vi "save.vi"(5 "Control Camera Properties 3":T2={"Packet Size"=1500, "Pixel Format"=17825797, "Gain in dB"=1.0, "Exposure Time in µs"=1500, "Stream Bytes per Second"=50000017} caption="Control Camera Properties" {"Stream Bytes per Second" min=1000000 max=124000000 step=100000 format="%.1p"; "Exposure Time in µs" min=21 max=153391689 format="%#.0f"; "Gain in dB" min=0.0 max=26.0 format="%#_2g"; "Pixel Format" items=["Mono 12 Packed"=17563654, "Mono 12"=17825797]}, 7 "Camera":T1, 8 "Path":path=path "C:/Users/loa/Documents/imaging-spectrometer/imaging-spectrometer/sub_vis/test", 9 "Complete File Name In":string, 10 "Array":u16[][](array[numeric]), 11 "reference":refnum<vi>) -> (0 "saving error out":errorcluster, 1 "Path out":path)   [LabVIEW 2014]
uses:
  type definitions/control camera properties.ctl
  <vilib>/Utility/file.llb/Write To Spreadsheet File (I64).vi
panel:
  # "Bytes"
  # "Trigger"
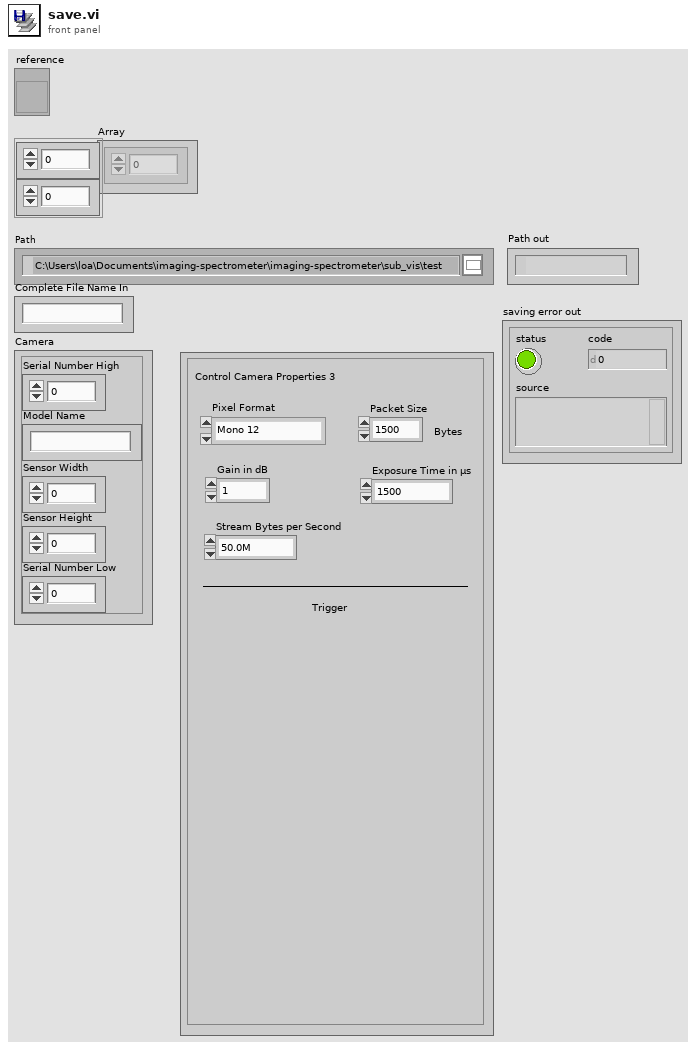
[diagram p1: front panel]
types:
  T1 = cluster{"Serial Number High":u32, "Model Name":string, "Sensor Width":u32, "Sensor Height":u32, "Serial Number Low":u32}
  T2 = typedef "control camera properties.ctl" = cluster{"Packet Size":u32, "Pixel Format":u32, "Gain in dB":dbl, "Exposure Time in µs":u32, "Stream Bytes per Second":u32}
  T3 = enum16{"open", "replace", "create", "open or create", "replace or create", "replace or create with confirmation"}
  T4 = typedef "imagedata.ctl" = cluster{"image type":i32, "image depth":i32, "image":u8[], "mask":u8[], "colors":u32[], "Rectangle":cluster{"left":i16, "top":i16, "right":i16, "bottom":i16}}
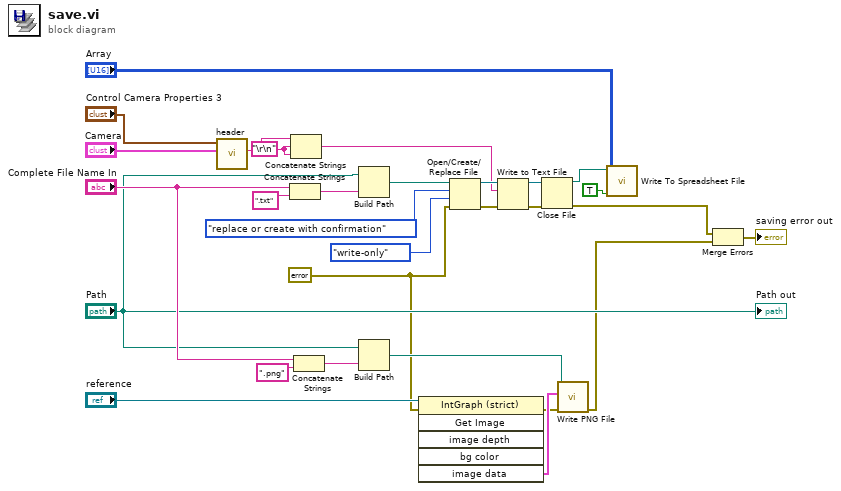
[diagram p0: block diagram]
diagram:
  w2 = errorcluster {"status"=FALSE, "code"=0, "source"=""} ("path error in")
  w14 = "\r\n"
  n1 = call "header.vi"("Camera"="Camera", "Control Camera Properties 3"="Control Camera Properties 3") -> ("Output string"=w15:string)  [unwired: 9 in]
  n2 = Concatenate Strings("Complete File Name In", ".txt" ("string")) -> (w19:string)
  n3 = Concatenate Strings(w15, w14, w14) -> (w13:string)
  n4 = Concatenate Strings("Complete File Name In", ".png" ("string")) -> (w17:string)
  n5 = Build Path(base path="Path", name or relative path=w19) -> (appended path=w21:path)
  n6 = Build Path(base path="Path", name or relative path=w17) -> (appended path=w29:path)
  n7 = invoke class="IntGraph (strict)" method="Get Image"(reference="reference", error in=w2) -> (error out=w6:errorcluster, "image data"=w16:T4)  [unwired: 4 in, 4 out]
  n8 = Open/Create/Replace File(file path (use dialog)=w21, error in=w2, operation (0:open)=T3."replace or create with confirmation", access (0:read/write)=enum16{"read/write", "read-only", "write-only"}."write-only") -> (refnum out=w25:refnum<file>, error out=w9:errorcluster)  [unwired: 2 in, 1 out]
  n9 = Write to Text File(file (use dialog)=w25, text=w13, error in=w9) -> (refnum out=w24:refnum<file>, error out=w8:errorcluster)  [unwired: 1 in, 1 out]
  n10 = Close File(refnum=w24, error in=w8) -> (path=w12:path, error out=w4:errorcluster)
  n11 = call <vilib>:"Write PNG File.vi"("error in (no error)"=w6, "image data"=w16, "path to PNG file"=w29) -> ("error out"=w3:errorcluster)  [unwired: 7 in, 1 out]
  n12 = call-poly <vilib>:"Write To Spreadsheet File.vi"("append to file? (new file:F)"=TRUE, "2D data"="Array", "file path (dialog if empty)"=w12) -> ()  [unwired: 5 in, 1 out]
  n13 = Merge Errors(w4, w3) -> (→"saving error out":errorcluster)
  "Path out" <- "Path"
